vi "tm3samp_05_functions.vi"() -> ()   [LabVIEW 2023]
panel:
  out "Image":u16[][](graph)
  in  "Snap":bool
  in  "Parameter":u32(ring)=4212128 items=["SENSOR MODE"=4212128, "READOUT SPEED"=4211872, "COLORTYPE"=4342960, "BIT PER CHANNEL"=4342976, "TRIGGER SOURCE"=1066144, "TRIGGER MODE"=1066400, "TRIGGER ACTIVE"=1066160, "TRIGGER GLOBAL EXPOSURE"=2049680, "TRIGGER POLARITY"=1066416, "TRIGGER TIMES"=1066448, "TRIGGER DELAY"=1066480, "EXPOSURE TIME CONTROL"=2049216, "EXPOSURE TIME"=2049184, "DEFECT CORRECT MODE"=4670368, "BINNING"=4215968, "SUBARRAY HPOS"=4220064, "SUBARRAY HSIZE"=4220080, "SUBARRAY VPOS"=4220096, "SUBARRAY VSIZE"=4220112, "SUBARRAY MODE"=4220128, "TIMING READOUT TIME"=4223904, "TIMING CYCLIC TRIGGER PERIOD"=4223920, "TIMING MIN TRIGGER BLANKING"=4223936, "TIMING MIN TRIGGER INTERVAL"=4223968, "TIMING GLOBAL EXPOSURE DELAY"=4224032, "TIMING EXPOSURE"=4223984, "TIMING INVALID EXPOSURE PERIOD"=4224000, "INTERNAL FRAME RATE"=4225952, "INTERNAL FRAME INTERVAL"=4225968, "FRAMEBUNDLE MODE"=4346784, "FRAMEBUNDLE NUMBER"=4346800, "FRAMEBUNDLE ROWBYTES"=4346816, "FRAMEBUNDLE FRAME STEP BYTES"=4346832, "IMAGE WIDTH"=4343200, "IMAGE HEIGHT"=4343216, "IMAGE ROWBYTES"=4343232, "IMAGE FRAMEBYTES"=4343248, "IMAGE TOP OFFSET BYTES"=4343264, "IMAGE PIXEL TYPE"=4343296, "IMAGE CAMERA STAMP"=4343440, "BUFFER ROWBYTES"=4343488, "BUFFER FRAMEBYTES"=4343504, "BUFFER TOP OFFSET BYTES"=4343520, "BUFFER PIXEL TYPE"=4343536, "RECORD FIXED BYTES PER FILE"=4343712, "RECORD FIXED BYTES PER SESSION"=4343728, "RECORD FIXED BYTES PER FRAME"=4343744, "NUMBER OF OUTPUT TRIGGER CONNECTOR"=1852320, "OUTPUT TRIGGER CHANNEL SYNC"=1852352, "OUTPUT TRIGGER PROGRAMABLE START"=1852384, "OUTPUT TRIGGER SOURCE[0]"=1852576, "OUTPUT TRIGGER POLARITY[0]"=1852592, "OUTPUT TRIGGER ACTIVE[0]"=1852608, "OUTPUT TRIGGER DELAY[0]"=1852624, "OUTPUT TRIGGER PERIOD[0]"=1852640, "OUTPUT TRIGGER KIND[0]"=1852656, "SYSTEM ALIVE"=16728992, "CONVERSION FACTOR COEFF"=16786336, "CONVERSION FACTOR OFFSET"=16786352, "IMAGE DETECTOR PIXEL WIDTH"=4344736, "IMAGE DETECTOR PIXEL HEIGHT"=4344752, "TIME STAMP PRODUCER"=4279712, "FRAME STAMP PRODUCER"=4279728]
  in  "Text Value":dbl(ring) items=["AREA"=1.0]
  in  "Value":dbl(slide) min=1.0 max=1.0 scale=0.9..1.0
  out "error out":errorcluster
  in  "stop":bool
  # "This example shows a way you can access\nmany of the functions available to the camera and see how they affect the captured image."
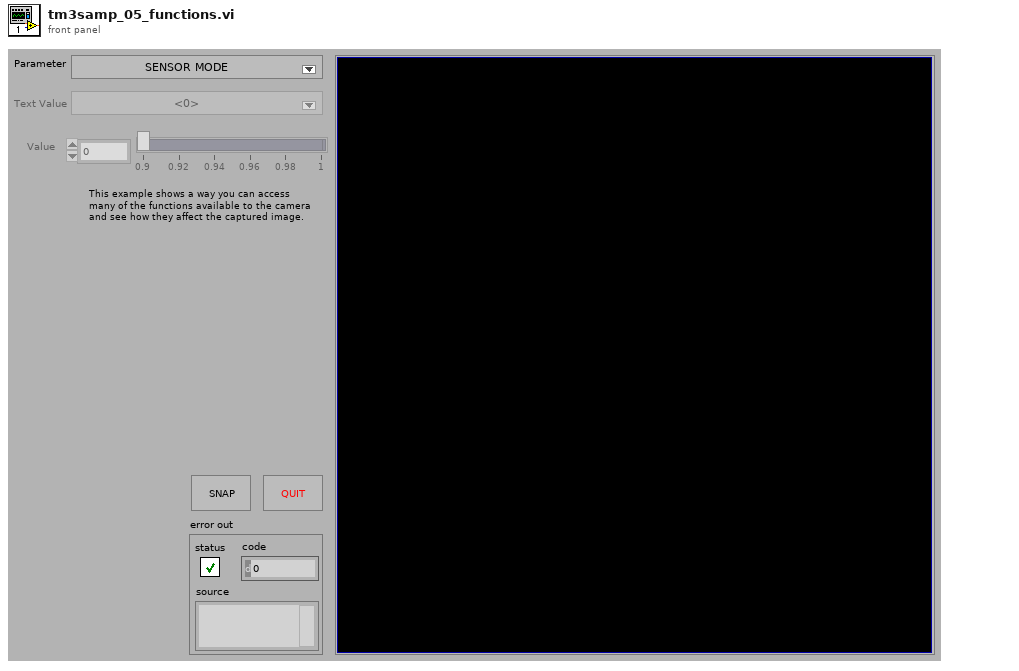
[diagram p1: front panel]
types:
  T1 = enum8{"Enabled", "Disabled", "Disabled and Grayed Out"}
  T2 = cluster{"Function Name":string, "Function ID":dbl}[]
  T3 = cluster{"Function Name":string, "Function ID":dbl}
  T4 = cluster{"height":u32, "width":u32, "datatype":u32}
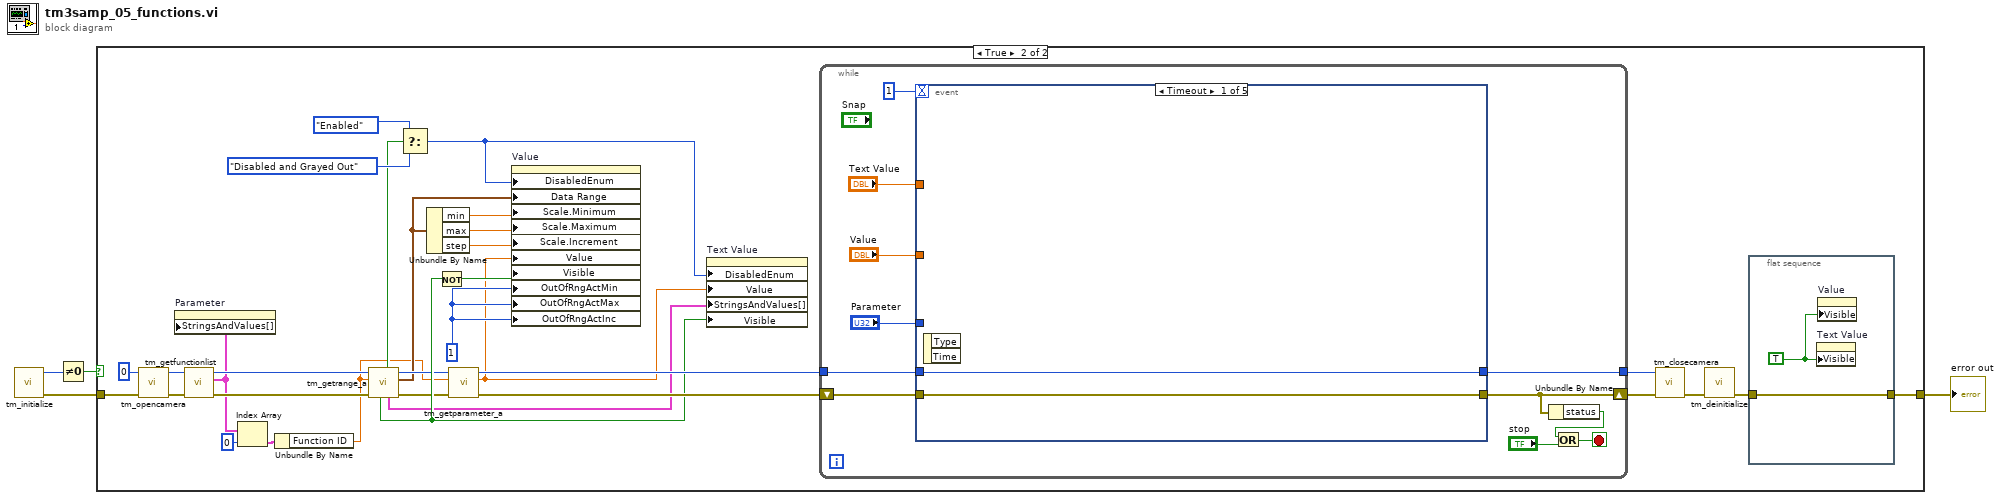
[diagram p0: block diagram]
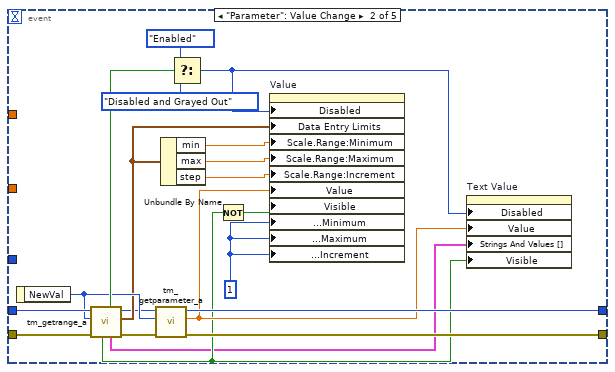
[diagram p3: hidden frame]
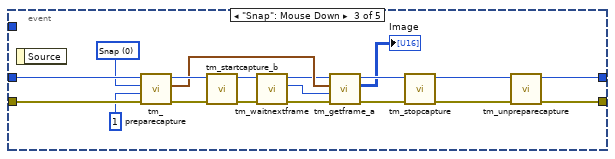
[diagram p4: hidden frame]
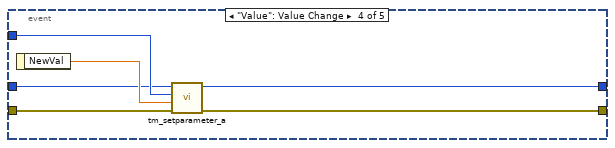
[diagram p5: hidden frame]
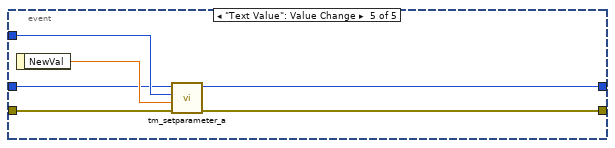
[diagram p6: hidden frame]
diagram:
  n1 = call "tm_initialize.vi"() -> ("error out"=w2:errorcluster, "Number Of Cameras"=w4:u32)  [unwired: 8 in, 2 out]
  n2 = Not Equal To 0?(x=w4) -> (x != 0?=w3:bool)
  n3 = case shown="True" w3 {
    tunnel: [w5 w32] -> w1
    tunnel: w2 -> [w5 w37]
    frame False {
    }
    frame True {
      w21 = u8 1 ("Out Of Range Action:Increment")
      n4 = call "tm_opencamera.vi"("error in (no error)"=w37, "Camera Index"=u32 0) -> ("error out"=w34:errorcluster, "Handle out"=w35:u32)  [unwired: 7 in, 1 out]
      n5 = call "tm_getfunctionlist.vi"("error in (no error)"=w34, "Handle in"=w35) -> ("error out"=w16:errorcluster, "Function List"=w9:T2, "Handle out"=w17:u32)  [unwired: 7 in]
      n6 = property on="Parameter" class="Ring (strict)"("StringsAndValues[]"=w9) -> ()  [unwired: 2 in, 2 out]
      n7 = Index Array(array=w9, index=0) -> (element=w7:T3)
      n8 = Unbundle By Name(w7) -> ("Function ID"=w6:dbl)
      n9 = call "tm_getrange_a.vi"("error in (no error)"=w16, "Parameter"=w6, "Handle in"=w17) -> ("error out"=w10:errorcluster, "Range"=w11:cluster{"min":dbl, "max":dbl, "step":dbl}, "Handle out"=w12:u32, "Value Names"=w14:cluster{"Name":string, "Value":dbl}[], "Writable"=w13:bool, "Text Values"=w15:bool)  [unwired: 2 in, 1 out]
      n10 = Select(t=T1."Enabled" ("Disabled"), s=w13, f=T1."Disabled and Grayed Out" ("Disabled")) -> (s? t:f=w26:T1)
      n11 = Unbundle By Name(w11) -> ("min"=w25:dbl, "max"=w24:dbl, "step"=w23:dbl)
      n12 = Not(x=w15) -> (.not. x?=w22:bool)
      n13 = call "tm_getparameter_a.vi"("error in (no error)"=w10, "Parameter"=w6, "Handle in"=w12) -> ("error out"=w18:errorcluster, "Value out"=w19:dbl, "Handle out"=w20:u32)  [unwired: 6 in]
      n14 = property on="Value" class="Slide (strict)"("DisabledEnum"=w26, "Data Range"=w11, "Scale.Minimum"=w25, "Scale.Maximum"=w24, "Scale.Increment"=w23, "Value"=w19, "Visible"=w22, "OutOfRngActMin"=w21, "OutOfRngActMax"=w21, "OutOfRngActInc"=w21) -> ()  [unwired: 2 in, 2 out]
      n15 = property on="Text Value" class="Ring (strict)"("DisabledEnum"=w26, "Value"=w19, "StringsAndValues[]"=w14, "Visible"=w15) -> ()  [unwired: 2 in, 2 out]
      n16 = while {
        tunnel: w20 -> [w46]
        tunnel: [w44] -> w30
        shift-right: [w43] -> w31
        shift-left: w18 -> [w47]
        stop <- w48 stop-if-true
        n17 = event shown="[0] Timeout" {
          selector: _ -> [_ _ _ _ _]
          dyn-events: _ -> [_ _ _ _ _]
          timeout: 1 -> [_ _ _ _ _]
          tunnel: w47 -> [w52 w59 w90 w97 w103]
          tunnel: w46 -> [w51 w60 w91 w94 w99]
          tunnel: [w51 w64 w80 w93 w98] -> w44
          tunnel: [w52 w62 w79 w92 w102] -> w43
          tunnel: "Parameter" -> [_ _ _ w95 w100]
          tunnel: "Value" -> [_ _ _ _ _]
          tunnel: "Text Value" -> [_ _ _ _ _]
          event Timeout {
            n18 = event-data() -> ()  [unwired: 1 in, 2 out]
          }
          event "Parameter": Value Change {
            w68 = u8 1 ("Out Of Range Action:Increment")
            n19 = event-data() -> ("NewVal"=w58:u32)  [unwired: 1 in]
            n20 = call "tm_getrange_a.vi"("error in (no error)"=w59, "Parameter"=w58, "Handle in"=w60) -> ("error out"=w55:errorcluster, "Range"=w54:cluster{"min":dbl, "max":dbl, "step":dbl}, "Handle out"=w53:u32, "Value Names"=w56:cluster{"Name":string, "Value":dbl}[], "Writable"=w61:bool, "Text Values"=w57:bool)  [unwired: 2 in, 1 out]
            n21 = call "tm_getparameter_a.vi"("error in (no error)"=w55, "Parameter"=w58, "Handle in"=w53) -> ("error out"=w62:errorcluster, "Value out"=w63:dbl, "Handle out"=w64:u32)  [unwired: 6 in]
            n22 = Unbundle By Name(w54) -> ("min"=w72:dbl, "max"=w71:dbl, "step"=w70:dbl)
            n23 = Select(t=T1."Enabled" ("Disabled"), s=w61, f=T1."Disabled and Grayed Out" ("Disabled")) -> (s? t:f=w67:T1)
            n24 = Not(x=w57) -> (.not. x?=w69:bool)
            n25 = property on="Value" class="Slide (strict)"("Disabled"=w67, "Data Entry Limits"=w54, "Scale.Range:Minimum"=w72, "Scale.Range:Maximum"=w71, "Scale.Range:Increment"=w70, "Value"=w63, "Visible"=w69, "Response to Value Outside Limits:Minimum"=w68, "Response to Value Outside Limits:Maximum"=w68, "Response to Value Outside Limits:Increment"=w68) -> ()  [unwired: 2 in, 2 out]
            n26 = property on="Text Value" class="Ring (strict)"("Disabled"=w67, "Value"=w63, "Strings And Values []"=w56, "Visible"=w57) -> ()  [unwired: 2 in, 2 out]
          }
          event "Snap": Mouse Down {
            w89 = 0 items=["Snap", "Sequence"] ("Capture mode")
            n27 = event-data() -> ()  [unwired: 1 in, 1 out]
            n28 = call "tm_preparecapture.vi"("error in (no error)"=w90, "Frames"=1, "Capture mode"=w89, "Handle in"=w91) -> ("error out"=w87:errorcluster, "Buffer Info"=w85:T4, "Handle out"=w86:u32)  [unwired: 4 in, 1 out]
            n29 = call "tm_startcapture_b.vi"("error in (no error)"=w87, "Handle in"=w86) -> ("error out"=w77:errorcluster, "Handle out"=w78:u32)  [unwired: 8 in]
            n30 = call "tm_waitnextframe.vi"("error in (no error)"=w77, "Handle in"=w78) -> ("error out"=w75:errorcluster, "Frame Index"=w74:i32, "Handle out"=w76:u32)  [unwired: 6 in, 1 out]
            n31 = call "tm_getframe_a.vi"("error in (no error)"=w75, "Frame Index"=w74, "Buffer Info"=w85, "Handle in"=w76) -> ("error out"=w83:errorcluster, "Data 16"=→"Image":u16[][], "Handle out"=w84:u32)  [unwired: 3 in, 2 out]
            n32 = call "tm_stopcapture.vi"("error in (no error)"=w83, "Handle in"=w84) -> ("error out"=w82:errorcluster, "Handle out"=w81:u32)  [unwired: 8 in]
            n33 = call "tm_unpreparecapture.vi"("error in (no error)"=w82, "Handle in"=w81) -> ("error out"=w79:errorcluster, "Handle out"=w80:u32)  [unwired: 8 in]
          }
          event "Value": Value Change {
            n34 = event-data() -> ("NewVal"=w96:dbl)  [unwired: 1 in]
            n35 = call "tm_setparameter_a.vi"("error in (no error)"=w97, "Value in"=w96, "Parameter"=w95, "Handle in"=w94) -> ("error out"=w92:errorcluster, "Handle out"=w93:u32)  [unwired: 6 in]
          }
          event "Text Value": Value Change {
            n36 = event-data() -> ("NewVal"=w101:dbl)  [unwired: 1 in]
            n37 = call "tm_setparameter_a.vi"("error in (no error)"=w103, "Value in"=w101, "Parameter"=w100, "Handle in"=w99) -> ("error out"=w102:errorcluster, "Handle out"=w98:u32)  [unwired: 6 in]
          }
        }
        n38 = Unbundle By Name(w43) -> ("status"=w49:bool)
        n39 = Or(x=w49, y="stop") -> (x .or. y?=w48:bool)
      }
      n40 = call "tm_closecamera.vi"("error in (no error)"=w31, "Handle in"=w30) -> ("error out"=w36:errorcluster)  [unwired: 9 in]
      n41 = call "tm_deinitialize.vi"("error in (no error)"=w36) -> ("error out"=w33:errorcluster)  [unwired: 10 in]
      n42 = flat-sequence {
        tunnel: w33 -> [w39]
        tunnel: [w39] -> w32
        frame #0 {
          w38 = TRUE
          n43 = property on="Text Value" class="Ring (strict)"("Visible"=w38) -> ()  [unwired: 2 in, 2 out]
          n44 = property on="Value" class="Slide (strict)"("Visible"=w38) -> ()  [unwired: 2 in, 2 out]
        }
      }
    }
  }
  "error out" <- w1
